vi "getCameraParameters.vi"(3 "Error IN":errorcluster, 5 "hCamera IN":u32) -> (0 "Error OUT":errorcluster, 1 "Camera Parameters":T2 {"Pixel Format" items=["PIXEL_FORMAT_MONO8", "PIXEL_FORMAT_MONO16", "PIXEL_FORMAT_YUV422", "PIXEL_FORMAT_BAYER8_GRBG", "PIXEL_FORMAT_BAYER16_GRBG", "PIXEL_FORMAT_RGB24", "PIXEL_FORMAT_RGB48", "PIXEL_FORMAT_BAYER8_RGGB", "PIXEL_FORMAT_BAYER8_GBRG ", "PIXEL_FORMAT_BAYER8_BGGR ", "PIXEL_FORMAT_BAYER16_RGGB ", "PIXEL_FORMAT_BAYER16_GBRG", "PIXEL_FORMAT_BAYER16_BGGR", "PIXEL_FORMAT_RGB32"]}, 2 "hCamera OUT":u32)   [LabVIEW 2010]
uses:
  <vilib>/addons/PixeLINK/Low Level Functions/CAMERA_FEATURES.llb/TDPU-CameraFeatures-PixelFormat.ctl
  <vilib>/addons/PixeLINK/Low Level Functions/CAMERA_FEATURES.llb/TDPU-CameraFeatures-FeatureIds.ctl
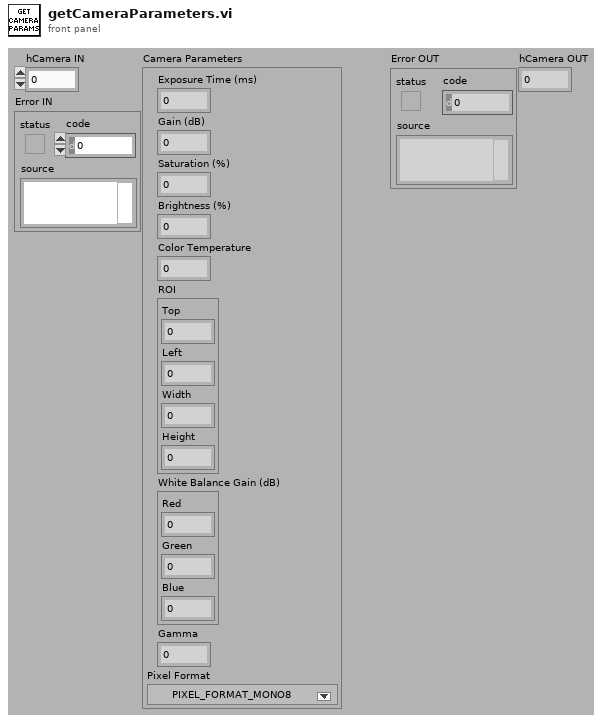
[diagram p1: front panel]
types:
  T1 = typedef "TDPU-CameraFeatures-PixelFormat.ctl" = u16
  T2 = cluster{"Exposure Time (ms)":dbl, "Gain (dB)":dbl, "Saturation (%)":dbl, "Brightness (%)":dbl, "Color Temperature":dbl, "ROI":cluster{"Top":i32, "Left":i32, "Width":i32, "Height":i32}, "White Balance Gain (dB)":cluster{"Red":dbl, "Green":dbl, "Blue":dbl}, "Gamma":dbl, "Pixel Format":T1}
  T3 = typedef "TDPU-CameraFeatures-FeatureIds.ctl" = u32
  T4 = cluster{"Top":i32, "Left":i32, "Width":i32, "Height":i32}
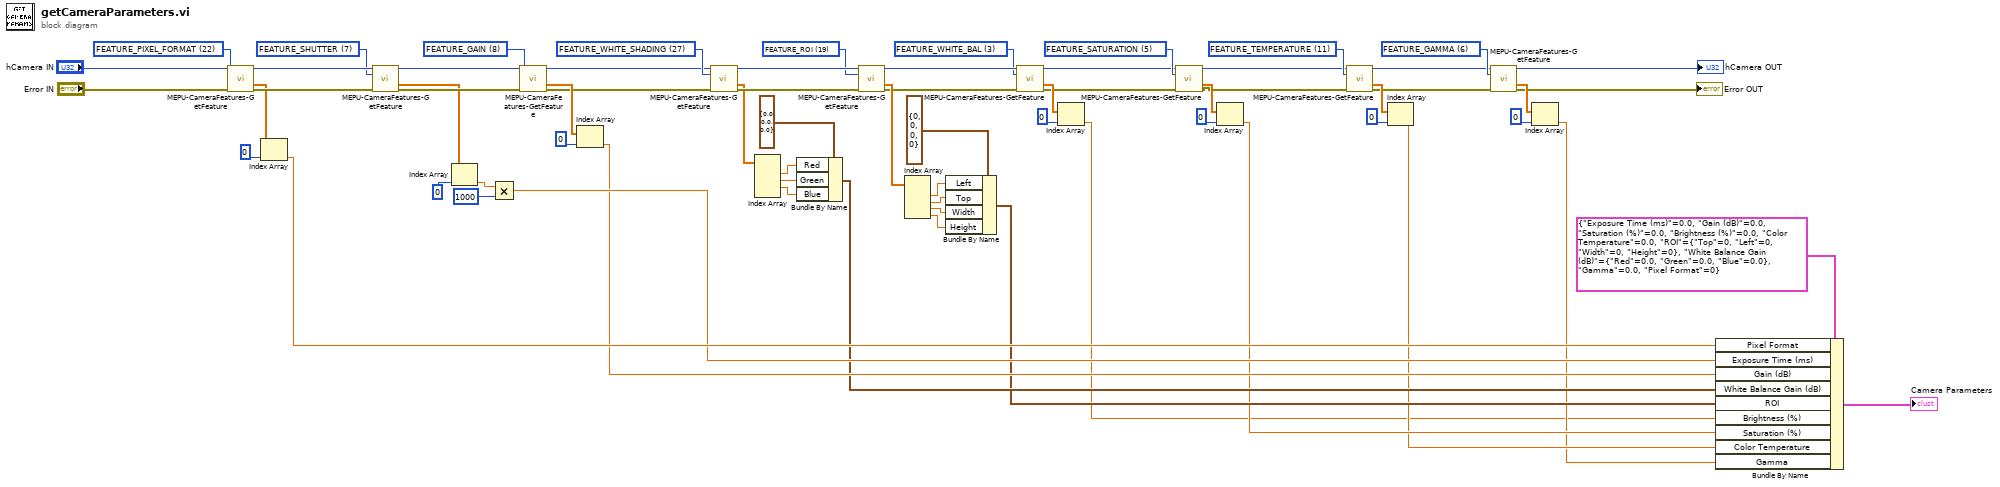
[diagram p0: block diagram]
diagram:
  w9 = T3 6 items=["FEATURE_BRIGHTNESS", "FEATURE_EXPOSURE", "FEATURE_SHARPNESS", "FEATURE_WHITE_BAL", "FEATURE_HUE", "FEATURE_SATURATION", "FEATURE_GAMMA", "FEATURE_SHUTTER", "FEATURE_GAIN", "FEATURE_IRIS", "FEATURE_FOCUS", "FEATURE_TEMPERATURE", "FEATURE_TRIGGER", "FEATURE_ZOOM", "FEATURE_PAN", "FEATURE_TILT", "FEATURE_OPT_FILTER", "FEATURE_GPIO", "FEATURE_FRAME_RATE", "FEATURE_ROI", "FEATURE_FLIP", "FEATURE_PIXEL_ADDRESSING", "FEATURE_PIXEL_FORMAT", "FEATURE_EXTENDED_SHUTTER", "FEATURE_AUTO_ROI", "FEATURE_LOOKUP_TABLE", "FEATURE_MEMORY_CHANNEL", "FEATURE_WHITE_SHADING", "FEATURE_ROTATE", "FEATURE_IMAGER_CLK_DIVISOR", "FEATURE_TRIG_WITH_CNTRLD_LIGHT", "FEATURE_MAX_PIXEL_SIZE"] ("uFeatureId IN")
  w18 = T3 11 items=["FEATURE_BRIGHTNESS", "FEATURE_EXPOSURE", "FEATURE_SHARPNESS", "FEATURE_WHITE_BAL", "FEATURE_HUE", "FEATURE_SATURATION", "FEATURE_GAMMA", "FEATURE_SHUTTER", "FEATURE_GAIN", "FEATURE_IRIS", "FEATURE_FOCUS", "FEATURE_TEMPERATURE", "FEATURE_TRIGGER", "FEATURE_ZOOM", "FEATURE_PAN", "FEATURE_TILT", "FEATURE_OPT_FILTER", "FEATURE_GPIO", "FEATURE_FRAME_RATE", "FEATURE_ROI", "FEATURE_FLIP", "FEATURE_PIXEL_ADDRESSING", "FEATURE_PIXEL_FORMAT", "FEATURE_EXTENDED_SHUTTER", "FEATURE_AUTO_ROI", "FEATURE_LOOKUP_TABLE", "FEATURE_MEMORY_CHANNEL", "FEATURE_WHITE_SHADING", "FEATURE_ROTATE", "FEATURE_IMAGER_CLK_DIVISOR", "FEATURE_TRIG_WITH_CNTRLD_LIGHT", "FEATURE_MAX_PIXEL_SIZE"] ("uFeatureId IN")
  w23 = T3 5 items=["FEATURE_BRIGHTNESS", "FEATURE_EXPOSURE", "FEATURE_SHARPNESS", "FEATURE_WHITE_BAL", "FEATURE_HUE", "FEATURE_SATURATION", "FEATURE_GAMMA", "FEATURE_SHUTTER", "FEATURE_GAIN", "FEATURE_IRIS", "FEATURE_FOCUS", "FEATURE_TEMPERATURE", "FEATURE_TRIGGER", "FEATURE_ZOOM", "FEATURE_PAN", "FEATURE_TILT", "FEATURE_OPT_FILTER", "FEATURE_GPIO", "FEATURE_FRAME_RATE", "FEATURE_ROI", "FEATURE_FLIP", "FEATURE_PIXEL_ADDRESSING", "FEATURE_PIXEL_FORMAT", "FEATURE_EXTENDED_SHUTTER", "FEATURE_AUTO_ROI", "FEATURE_LOOKUP_TABLE", "FEATURE_MEMORY_CHANNEL", "FEATURE_WHITE_SHADING", "FEATURE_ROTATE", "FEATURE_IMAGER_CLK_DIVISOR", "FEATURE_TRIG_WITH_CNTRLD_LIGHT", "FEATURE_MAX_PIXEL_SIZE"] ("uFeatureId IN")
  w27 = T3 3 items=["FEATURE_BRIGHTNESS", "FEATURE_EXPOSURE", "FEATURE_SHARPNESS", "FEATURE_WHITE_BAL", "FEATURE_HUE", "FEATURE_SATURATION", "FEATURE_GAMMA", "FEATURE_SHUTTER", "FEATURE_GAIN", "FEATURE_IRIS", "FEATURE_FOCUS", "FEATURE_TEMPERATURE", "FEATURE_TRIGGER", "FEATURE_ZOOM", "FEATURE_PAN", "FEATURE_TILT", "FEATURE_OPT_FILTER", "FEATURE_GPIO", "FEATURE_FRAME_RATE", "FEATURE_ROI", "FEATURE_FLIP", "FEATURE_PIXEL_ADDRESSING", "FEATURE_PIXEL_FORMAT", "FEATURE_EXTENDED_SHUTTER", "FEATURE_AUTO_ROI", "FEATURE_LOOKUP_TABLE", "FEATURE_MEMORY_CHANNEL", "FEATURE_WHITE_SHADING", "FEATURE_ROTATE", "FEATURE_IMAGER_CLK_DIVISOR", "FEATURE_TRIG_WITH_CNTRLD_LIGHT", "FEATURE_MAX_PIXEL_SIZE"] ("uFeatureId IN")
  w42 = T3 19 items=["FEATURE_BRIGHTNESS", "FEATURE_EXPOSURE", "FEATURE_SHARPNESS", "FEATURE_WHITE_BAL", "FEATURE_HUE", "FEATURE_SATURATION", "FEATURE_GAMMA", "FEATURE_SHUTTER", "FEATURE_GAIN", "FEATURE_IRIS", "FEATURE_FOCUS", "FEATURE_TEMPERATURE", "FEATURE_TRIGGER", "FEATURE_ZOOM", "FEATURE_PAN", "FEATURE_TILT", "FEATURE_OPT_FILTER", "FEATURE_GPIO", "FEATURE_FRAME_RATE", "FEATURE_ROI", "FEATURE_FLIP", "FEATURE_PIXEL_ADDRESSING", "FEATURE_PIXEL_FORMAT", "FEATURE_EXTENDED_SHUTTER", "FEATURE_AUTO_ROI", "FEATURE_LOOKUP_TABLE", "FEATURE_MEMORY_CHANNEL", "FEATURE_WHITE_SHADING", "FEATURE_ROTATE", "FEATURE_IMAGER_CLK_DIVISOR", "FEATURE_TRIG_WITH_CNTRLD_LIGHT", "FEATURE_MAX_PIXEL_SIZE"] ("uFeatureId IN")
  w52 = T3 27 items=["FEATURE_BRIGHTNESS", "FEATURE_EXPOSURE", "FEATURE_SHARPNESS", "FEATURE_WHITE_BAL", "FEATURE_HUE", "FEATURE_SATURATION", "FEATURE_GAMMA", "FEATURE_SHUTTER", "FEATURE_GAIN", "FEATURE_IRIS", "FEATURE_FOCUS", "FEATURE_TEMPERATURE", "FEATURE_TRIGGER", "FEATURE_ZOOM", "FEATURE_PAN", "FEATURE_TILT", "FEATURE_OPT_FILTER", "FEATURE_GPIO", "FEATURE_FRAME_RATE", "FEATURE_ROI", "FEATURE_FLIP", "FEATURE_PIXEL_ADDRESSING", "FEATURE_PIXEL_FORMAT", "FEATURE_EXTENDED_SHUTTER", "FEATURE_AUTO_ROI", "FEATURE_LOOKUP_TABLE", "FEATURE_MEMORY_CHANNEL", "FEATURE_WHITE_SHADING", "FEATURE_ROTATE", "FEATURE_IMAGER_CLK_DIVISOR", "FEATURE_TRIG_WITH_CNTRLD_LIGHT", "FEATURE_MAX_PIXEL_SIZE"] ("uFeatureId IN")
  w65 = T3 8 items=["FEATURE_BRIGHTNESS", "FEATURE_EXPOSURE", "FEATURE_SHARPNESS", "FEATURE_WHITE_BAL", "FEATURE_HUE", "FEATURE_SATURATION", "FEATURE_GAMMA", "FEATURE_SHUTTER", "FEATURE_GAIN", "FEATURE_IRIS", "FEATURE_FOCUS", "FEATURE_TEMPERATURE", "FEATURE_TRIGGER", "FEATURE_ZOOM", "FEATURE_PAN", "FEATURE_TILT", "FEATURE_OPT_FILTER", "FEATURE_GPIO", "FEATURE_FRAME_RATE", "FEATURE_ROI", "FEATURE_FLIP", "FEATURE_PIXEL_ADDRESSING", "FEATURE_PIXEL_FORMAT", "FEATURE_EXTENDED_SHUTTER", "FEATURE_AUTO_ROI", "FEATURE_LOOKUP_TABLE", "FEATURE_MEMORY_CHANNEL", "FEATURE_WHITE_SHADING", "FEATURE_ROTATE", "FEATURE_IMAGER_CLK_DIVISOR", "FEATURE_TRIG_WITH_CNTRLD_LIGHT", "FEATURE_MAX_PIXEL_SIZE"] ("uFeatureId IN")
  w60 = T3 7 items=["FEATURE_BRIGHTNESS", "FEATURE_EXPOSURE", "FEATURE_SHARPNESS", "FEATURE_WHITE_BAL", "FEATURE_HUE", "FEATURE_SATURATION", "FEATURE_GAMMA", "FEATURE_SHUTTER", "FEATURE_GAIN", "FEATURE_IRIS", "FEATURE_FOCUS", "FEATURE_TEMPERATURE", "FEATURE_TRIGGER", "FEATURE_ZOOM", "FEATURE_PAN", "FEATURE_TILT", "FEATURE_OPT_FILTER", "FEATURE_GPIO", "FEATURE_FRAME_RATE", "FEATURE_ROI", "FEATURE_FLIP", "FEATURE_PIXEL_ADDRESSING", "FEATURE_PIXEL_FORMAT", "FEATURE_EXTENDED_SHUTTER", "FEATURE_AUTO_ROI", "FEATURE_LOOKUP_TABLE", "FEATURE_MEMORY_CHANNEL", "FEATURE_WHITE_SHADING", "FEATURE_ROTATE", "FEATURE_IMAGER_CLK_DIVISOR", "FEATURE_TRIG_WITH_CNTRLD_LIGHT", "FEATURE_MAX_PIXEL_SIZE"] ("uFeatureId IN")
  w53 = T3 22 items=["FEATURE_BRIGHTNESS", "FEATURE_EXPOSURE", "FEATURE_SHARPNESS", "FEATURE_WHITE_BAL", "FEATURE_HUE", "FEATURE_SATURATION", "FEATURE_GAMMA", "FEATURE_SHUTTER", "FEATURE_GAIN", "FEATURE_IRIS", "FEATURE_FOCUS", "FEATURE_TEMPERATURE", "FEATURE_TRIGGER", "FEATURE_ZOOM", "FEATURE_PAN", "FEATURE_TILT", "FEATURE_OPT_FILTER", "FEATURE_GPIO", "FEATURE_FRAME_RATE", "FEATURE_ROI", "FEATURE_FLIP", "FEATURE_PIXEL_ADDRESSING", "FEATURE_PIXEL_FORMAT", "FEATURE_EXTENDED_SHUTTER", "FEATURE_AUTO_ROI", "FEATURE_LOOKUP_TABLE", "FEATURE_MEMORY_CHANNEL", "FEATURE_WHITE_SHADING", "FEATURE_ROTATE", "FEATURE_IMAGER_CLK_DIVISOR", "FEATURE_TRIG_WITH_CNTRLD_LIGHT", "FEATURE_MAX_PIXEL_SIZE"] ("uFeatureId IN")
  n1 = call <vilib>:"MEPU-CameraFeatures-GetFeature.vi"("hCamera IN"="hCamera IN", "uFeatureId IN"=w53, "Error IN"="Error IN") -> ("hCamera OUT"=w62:u32, "pParms OUT"=w54:dbl[], "Error OUT"=w61:errorcluster)  [unwired: 8 in, 2 out]
  n2 = Index Array(array=w54, index=0) -> (element=w47:dbl)
  n3 = call <vilib>:"MEPU-CameraFeatures-GetFeature.vi"("hCamera IN"=w62, "uFeatureId IN"=w60, "Error IN"=w61) -> ("hCamera OUT"=w64:u32, "pParms OUT"=w59:dbl[], "Error OUT"=w63:errorcluster)  [unwired: 8 in, 2 out]
  n4 = Index Array(array=w59, index=0) -> (element=w56:dbl)
  n5 = Multiply(x=w56, y=1000) -> (x*y=w46:dbl)
  n6 = call <vilib>:"MEPU-CameraFeatures-GetFeature.vi"("hCamera IN"=w64, "uFeatureId IN"=w65, "Error IN"=w63) -> ("hCamera OUT"=w51:u32, "pParms OUT"=w67:dbl[], "Error OUT"=w50:errorcluster)  [unwired: 8 in, 2 out]
  n7 = Index Array(array=w67, index=0) -> (element=w45:dbl)
  n8 = call <vilib>:"MEPU-CameraFeatures-GetFeature.vi"("hCamera IN"=w51, "uFeatureId IN"=w52, "Error IN"=w50) -> ("hCamera OUT"=w44:u32, "pParms OUT"=w35:dbl[], "Error OUT"=w43:errorcluster)  [unwired: 8 in, 2 out]
  n9 = Index Array(array=w35) -> (element #1=w33:dbl, element #2=w32:dbl, element #3=w31:dbl)  [unwired: 4 in, 1 out]
  n10 = Bundle By Name(cluster=cluster{"Red":dbl, "Green":dbl, "Blue":dbl} {"Red"=0.0, "Green"=0.0, "Blue"=0.0} ("White Balance Gain (dB)"), "Red"=w33, "Green"=w32, "Blue"=w31) -> (w30:cluster{"Red":dbl, "Green":dbl, "Blue":dbl})
  n11 = call <vilib>:"MEPU-CameraFeatures-GetFeature.vi"("hCamera IN"=w44, "uFeatureId IN"=w42, "Error IN"=w43) -> ("hCamera OUT"=w28:u32, "pParms OUT"=w40:dbl[], "Error OUT"=w29:errorcluster)  [unwired: 8 in, 2 out]
  n12 = Index Array(array=w40) -> (element #1=w39:dbl, element #2=w38:dbl, element #3=w37:dbl, element #4=w36:dbl)  [unwired: 4 in]
  n13 = Bundle By Name(cluster=T4 {"Top"=0, "Left"=0, "Width"=0, "Height"=0} ("ROI"), "Left"=w39, "Top"=w38, "Width"=w37, "Height"=w36) -> (w24:T4)
  n14 = call <vilib>:"MEPU-CameraFeatures-GetFeature.vi"("hCamera IN"=w28, "uFeatureId IN"=w27, "Error IN"=w29) -> ("hCamera OUT"=w20:u32, "pParms OUT"=w25:dbl[], "Error OUT"=w19:errorcluster)  [unwired: 8 in, 2 out]
  n15 = Index Array(array=w25, index=0) -> (element=w1:dbl)
  n16 = call <vilib>:"MEPU-CameraFeatures-GetFeature.vi"("hCamera IN"=w20, "uFeatureId IN"=w23, "Error IN"=w19) -> ("hCamera OUT"=w15:u32, "pParms OUT"=w21:dbl[], "Error OUT"=w14:errorcluster)  [unwired: 8 in, 2 out]
  n17 = Index Array(array=w21, index=0) -> (element=w13:dbl)
  n18 = call <vilib>:"MEPU-CameraFeatures-GetFeature.vi"("hCamera IN"=w15, "uFeatureId IN"=w18, "Error IN"=w14) -> ("hCamera OUT"=w5:u32, "pParms OUT"=w16:dbl[], "Error OUT"=w8:errorcluster)  [unwired: 8 in, 2 out]
  n19 = Index Array(array=w16, index=0) -> (element=w12:dbl)
  n20 = call <vilib>:"MEPU-CameraFeatures-GetFeature.vi"("hCamera IN"=w5, "uFeatureId IN"=w9, "Error IN"=w8) -> ("hCamera OUT"=→"hCamera OUT":u32, "pParms OUT"=w10:dbl[], "Error OUT"=→"Error OUT":errorcluster)  [unwired: 8 in, 2 out]
  n21 = Index Array(array=w10, index=0) -> (element=w4:dbl)
  n22 = Bundle By Name(cluster=T2 {"Exposure Time (ms)"=0.0, "Gain (dB)"=0.0, "Saturation (%)"=0.0, "Brightness (%)"=0.0, "Color Temperature"=0.0, "ROI"={"Top"=0, "Left"=0, "Width"=0, "Height"=0}, "White Balance Gain (dB)"={"Red"=0.0, "Green"=0.0, "Blue"=0.0}, "Gamma"=0.0, "Pixel Format"=0} ("Camera Parameters"), "Pixel Format"=w47, "Exposure Time (ms)"=w46, "Gain (dB)"=w45, "White Balance Gain (dB)"=w30, "ROI"=w24, "Brightness (%)"=w1, "Saturation (%)"=w13, "Color Temperature"=w12, "Gamma"=w4) -> (→"Camera Parameters":T2)
